vi "TCP AK-LNI Antwort empfangen.vi"(8 "Fehler (Eingang)":errorcluster, 11 "Verbindungs-ID":refnum<k5>) -> (0 "Fehler (Ausgang)":errorcluster, 1 "ES (Error Status)":string, 2 "Daten":string, 3 "Verbindungs-ID":refnum<k5>, 4 "Lesepuffer":string, 5 "Befehl":string)   [LabVIEW 2020, in "Linearisierung v2.lvlib" / "Gasteiler.lvlib" / "AK Komm Gasteiler.lvlib"]
doc: "Liest die Anwort auf einen AK-Befehl von der COM-Schnittstelle und wertet die Telegrammteile aus:\n\nBefehl: Wiederholung des gesendeten Befehls, Ausnahme ???? ... Befehl unbekannt\nDaten: Daten (String)\nES: Error Status (String), 0..kein Fehler\n\nDer ErrorStatus wird ausgewertet und liefert im Fehlercluster \"Fehler(Ausgang)\" die Fehlerursache in Klartext."
uses:
  AK Komm Gasteiler.lvlib
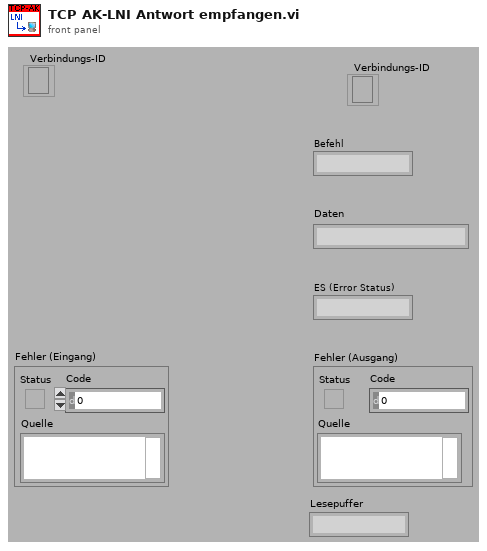
[diagram p1: front panel]
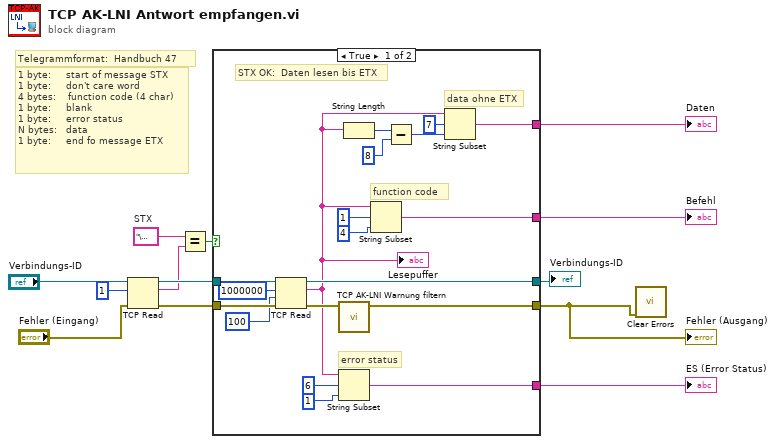
[diagram p0: block diagram]
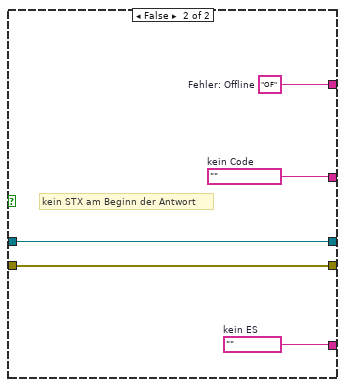
[diagram p2: hidden frame]
diagram:
  w9 = "\u0002"  # STX
  # "Telegrammformat:  Handbuch 47"
  # "1 byte:     start of message STX\n1 byte:     don't care word\n4 bytes:    function code (4 char)\n1 byte:     blank\n1 byte:     error status\nN bytes:   data\n1 byte:     end fo message ETX"
  n1 = TCP Read(connection ID="Verbindungs-ID", bytes to read=u32 1 ("Byte-Anzahl"), error in (no error)="Fehler (Eingang)") -> (connection ID out=w11:refnum<k5>, data out=w6:string, error out=w10:errorcluster)  [unwired: 2 in]
  n2 = Equal?(x=w9, y=w6) -> (x = y?=w7:bool)
  n3 = case shown="True" w7 {
    tunnel: w11 -> [w32 w37]
    tunnel: w10 -> [w31 w36]
    tunnel: [w28 w37] -> w1
    tunnel: [w27 w36] -> w2
    tunnel: [w15 w33] -> w8
    tunnel: [w17 w35] -> w5
    tunnel: [w16 w34] -> w4
    frame True {
      # "error status"
      # "function code"
      # "data ohne ETX"
      # "STX OK:  Daten lesen bis ETX"
      n4 = TCP Read(connection ID=w32, bytes to read=u32 1000000 ("Byte-Anzahl"), error in (no error)=w31, 9:100 ("Timeout in ms (25000)")) -> (connection ID out=w28:refnum<k5>, data out=w18:string, error out=w29:errorcluster)  [unwired: 1 in]
      "Lesepuffer" <- w18
      n5 = call "TCP AK-LNI Warnung filtern.vi"("error in (no error)"=w29) -> ("error out"=w27:errorcluster)  [unwired: 10 in]
      n6 = String Subset(string=w18, offset (0)=6 ("Offset (0)"), length (rest)=1 ("Länge (Rest)")) -> (substring=w16:string)
      n7 = String Length(string=w18) -> (length=w26:i32)
      n8 = String Subset(string=w18, offset (0)=1 ("Offset (0)"), length (rest)=4 ("Länge (Rest)")) -> (substring=w17:string)
      n9 = Subtract(x=w26, y=8) -> (x-y=w24:i32)
      n10 = String Subset(string=w18, offset (0)=7 ("Offset (0)"), length (rest)=w24) -> (substring=w15:string)
    }
    frame False {
      w33 = "OF"  # Fehler: Offline
      w34 = ""  # kein ES
      w35 = ""  # kein Code
      # "kein STX am Beginn der Antwort"
    }
  }
  "Fehler (Ausgang)" <- w2
  "Daten" <- w8
  "Befehl" <- w5
  "ES (Error Status)" <- w4
  "Verbindungs-ID" <- w1
  n11 = call <vilib>:"Clear Errors.vi"("error in (no error)"=w2) -> ()  [unwired: 5 in, 2 out]
